vi "Write WS URI.vi"(8 "error in (no error)":errorcluster, 10 "WS URI":string, 11 "WebSocket Client in":refnum<class "WebSocket Client.lvclass">) -> (0 "error out":errorcluster, 3 "WebSocket Client out":refnum<class "WebSocket Client.lvclass">)   [LabVIEW 2017, in "WebSocket Actors.lvlib" / "WebSocket Client.lvclass"]
uses:
  WebSocket Client.lvclass
  C:/Projects/Shared Libraries/WebSocket Actor/WebSocket Actor/WebSocket Connection/WebSocket Connection.lvclass
  WebSocket Client.lvclass/WebSocket Client.ctl
  Websockets/LV WebSockets.lvlib
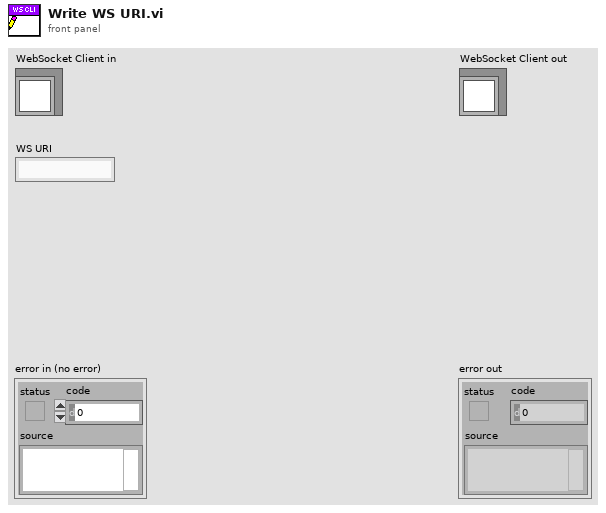
[diagram p1: front panel]
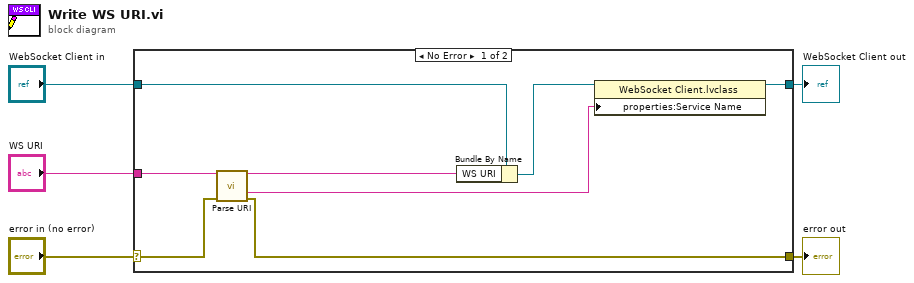
[diagram p0: block diagram]
diagram:
  n1 = case shown="No Error" "error in (no error)" {
    selector: "error in (no error)" -> [w10 w14]
    tunnel: [w9 w14] -> w4
    tunnel: [w7 w15] -> w2
    tunnel: "WebSocket Client in" -> [w13 w15]
    tunnel: "WS URI" -> [w11 _]
    frame No Error {
      n2 = call "Parse URI.vi"("URI"=w11, "error in"=w10) -> ("URI Out"=w8:string, "Resource Name"=w6:string, "error out"=w9:errorcluster)  [unwired: 7 in, 4 out]
      n3 = Bundle By Name(cluster=w13, "WS URI"=w8) -> (w12:refnum<class "WebSocket Client.lvclass">)
      n4 = property class="WebSocket Client.lvclass"(reference=w12, "properties:Service Name"=w6) -> (reference out=w7:refnum<class "WebSocket Client.lvclass">)  [unwired: 1 in, 1 out]
    }
    frame Error {
    }
  }
  "error out" <- w4
  "WebSocket Client out" <- w2
